vi "get ID.vi"(11 "task in":refnum<class "task.lvclass">) -> (2 "ID":string, 3 "task out":refnum<class "task.lvclass">)   [LabVIEW 2013, in "task.lvclass"]
uses:
  task.lvclass
  task.lvclass/task.ctl
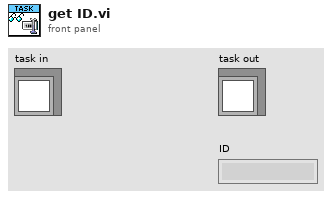
[diagram p1: front panel]
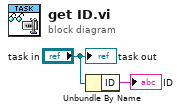
[diagram p0: block diagram]
diagram:
  n1 = Unbundle By Name("task in") -> ("ID"=→"ID":string)
  "task out" <- "task in"
